vi "Match True & False StringPart 8.vi"() -> ()   [LabVIEW 2020]
panel:
  out "selection":bool
  out "output string":string
  in  "string":string
  # "Match True/False String"
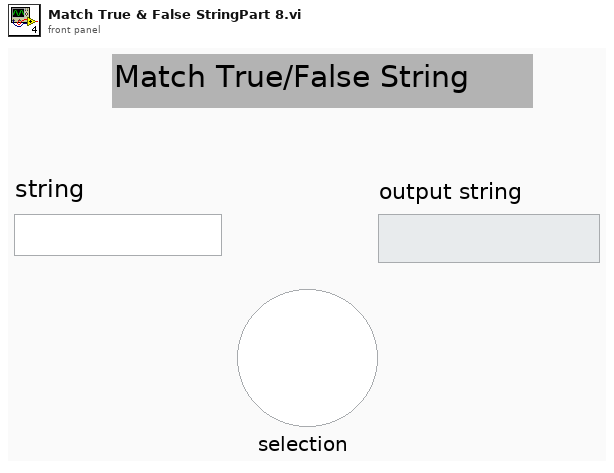
[diagram p1: front panel]
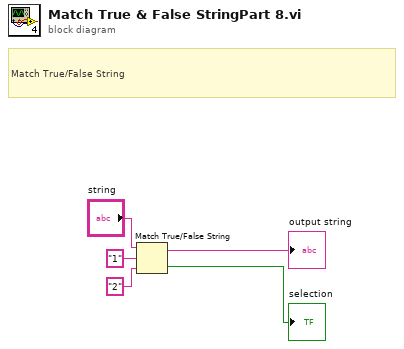
[diagram p0: block diagram]
diagram:
  # "Match True/False String"
  n1 = Match True/False String(2:"2" ("false string"), 3:"1" ("true string"), 4:"string") -> (0:→"selection":bool, 1:→"output string":string)
